vi "Deviated Result.vi"(8 "Error in":errorcluster, 11 "DAC in":refnum<class "DAC.lvclass">) -> (0 "Error out":errorcluster, 3 "DAC out":refnum<class "DAC.lvclass">)   [LabVIEW 2020, in "DAC.lvclass"]
doc: "Generates deviated values for DAC"
uses:
  DAC.lvclass
  D:/SDLC/Class/INL DNL Test/Device/Parent/Device.lvclass
  <vilib>/numeric/Random Number (Range) DBL.vi
  DAC.lvclass/DAC.ctl
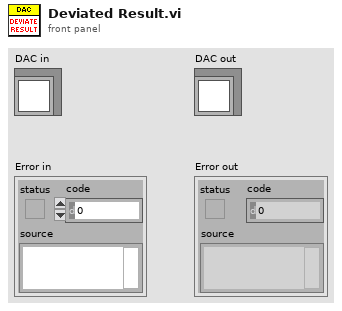
[diagram p1: front panel]
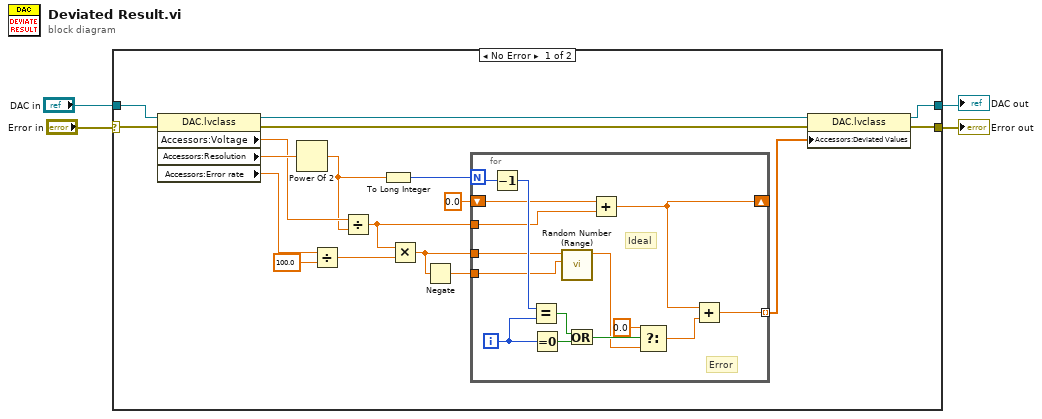
[diagram p0: block diagram]
diagram:
  n1 = case shown="No Error" "Error in" {
    selector: "Error in" -> [w22 w39]
    tunnel: [w8 w39] -> w3
    tunnel: "DAC in" -> [w21 w38]
    tunnel: [w7 w38] -> w1
    frame No Error {
      n2 = property class="DAC.lvclass"(reference=w21, error in=w22) -> (reference out=w11:refnum<class "DAC.lvclass">, error out=w10:errorcluster, "Accessors:Voltage"=w19:dbl, "Accessors:Resolution"=w20:dbl, "Accessors:Error rate"=w18:dbl)
      n3 = Power Of 2(x=w20) -> (2^x=w6:dbl)
      n4 = Divide(x=w18, y=100.0) -> (x/y=w16:dbl)
      n5 = Divide(x=w19, y=w6) -> (x/y=w13:dbl)
      n6 = To Long Integer(number=w6) -> (32bit integer=w5:i32)
      n7 = Multiply(x=w13, y=w16) -> (x*y=w14:dbl)
      n8 = Negate(x=w14) -> (-x=w15:dbl)
      n9 = for {
        N: w5 -> [w35]
        tunnel: w14 -> [w31]
        tunnel: w15 -> [w29]
        tunnel: w13 -> [w28]
        shift-right: [w25] -> _
        shift-left: 0.0 -> [w27]
        tunnel: [w24] -> w9 mode=indexing
        i -> [w36]
        # "Error"
        # "Ideal"
        n10 = Decrement(x=w35) -> (x-1=w34:i32)
        n11 = Equal?(x=w34, y=w36) -> (x = y?=w33:bool)
        n12 = Equal To 0?(x=w36) -> (x = 0?=w37:bool)
        n13 = call-poly <vilib>:"Random Number (Range).vi"("lower bound (0)"=w29, "upper bound (100)"=w31) -> ("number"=w23:dbl)  [unwired: 9 in]
        n14 = Or(x=w33, y=w37) -> (x .or. y?=w32:bool)
        n15 = Add(x=w27, y=w28) -> (x+y=w25:dbl)
        n16 = Select(t=0.0, s=w32, f=w23) -> (s? t:f=w26:dbl)
        n17 = Add(x=w25, y=w26) -> (x+y=w24:dbl)
      }
      n18 = property class="DAC.lvclass"(reference=w11, error in=w10, "Accessors:Deviated Values"=w9) -> (reference out=w7:refnum<class "DAC.lvclass">, error out=w8:errorcluster)
    }
    frame Error {
    }
  }
  "Error out" <- w3
  "DAC out" <- w1
